vi "Write Seconds Before Showing.vi"(8 "error in (no error)":errorcluster, 10 "Seconds Before Showing":dbl, 11 "MGI_Progress Bar Options in":refnum<class "Progress Bar Settings.lvclass">) -> (0 "error out":errorcluster, 3 "MGI_Progress Bar Options out":refnum<class "Progress Bar Settings.lvclass">)   [LabVIEW 2016, in "Progress Bar Settings.lvclass"]
uses:
  <userlib>/_MGI/User Interface/Progress Bar/Progress Bar Settings/Progress Bar Settings.lvclass
  <userlib>/_MGI/User Interface/Progress Bar/Progress Bar Settings/Progress Bar Settings.lvclass/Progress Bar Settings.ctl
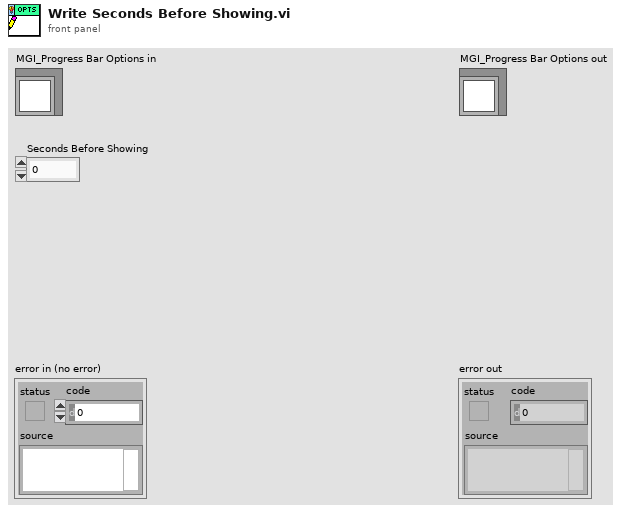
[diagram p1: front panel]
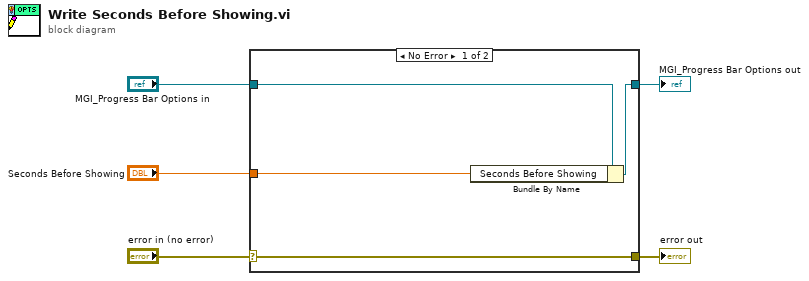
[diagram p0: block diagram]
diagram:
  n1 = case shown="No Error" "error in (no error)" {
    selector: "error in (no error)" -> [w9 w10]
    tunnel: [w9 w10] -> w4
    tunnel: [w7 w11] -> w2
    tunnel: "MGI_Progress Bar Options in" -> [w8 w11]
    tunnel: "Seconds Before Showing" -> [w6 _]
    frame No Error {
      n2 = Bundle By Name(cluster=w8, "Seconds Before Showing"=w6) -> (w7:refnum<class "Progress Bar Settings.lvclass">)
    }
    frame Error {
    }
  }
  "error out" <- w4
  "MGI_Progress Bar Options out" <- w2
